vi "TraceViewer.vi"   [LabVIEW 2013]
uses:
  Dispatcher/Dispatcher.lvclass
  <vilib>/ActorFramework/Message Queue/Message Queue.lvclass/Message Queue.ctl
  <vilib>/ActorFramework/Actor/Actor.lvclass
  <vilib>/ActorFramework/Message Queue/Message Queue.lvclass
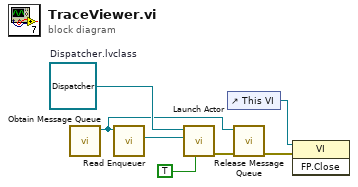
[diagram p0: block diagram]
diagram:
  w6 = refnum<class "Dispatcher.lvclass"> refnum  # Dispatcher.lvclass
  n1 = call <vilib>:"Obtain Message Queue.vi"() -> ("Message Queue"=w3:refnum<class "Message Queue.lvclass">)  [unwired: 10 in, 1 out]
  n2 = call <vilib>:"Read Enqueuer.vi"("Message Queue"=w3) -> ("Message Enqueuer"=w7:refnum<class "Message Enqueuer.lvclass">)  [unwired: 10 in]
  n3 = call <vilib>:"Launch Actor.vi"("Open Actor Core front panel? (F)"=TRUE, "Actor-to-Caller Enqueuer"=w7, "Actor"=w6) -> ("error out"=w4:errorcluster)  [unwired: 7 in, 1 out]
  n4 = control-ref of="This VI"() -> (w2:refnum<vi>)
  n5 = call <vilib>:"Release Message Queue.vi"("error in (no error)"=w4, "Message Queue"=w3) -> ("error out"=w1:errorcluster)  [unwired: 8 in, 1 out]
  n6 = invoke class="VI" method="FP.Close"(reference=w2, error in=w1) -> ()  [unwired: 1 in, 3 out]
